vi "Get Sciscan Scope Image Equalization.vi"(0 "GFG Refnum":refnum<vi>, 5 "error in":errorcluster) -> (14 "GFG Refnum Out":refnum<vi>, 15 "Green Channel":cluster{dbl, dbl}(slide)={0.0, 7.070707070707071} caption="Green Channel Equalizer" scale=-32768.0..32767.0, 16 "Auto Adjust Green":bool, 17 "Red Channel":cluster{dbl, dbl}(slide)={0.0, 7.070707070707071} caption="Green Channel Equalizer" scale=-32768.0..32767.0, 18 "Auto Adjust Red":bool, 19 "error out":errorcluster)   [LabVIEW 2012, in "Sciscan Scope Daemon.lvlib"]
uses:
  Sciscan Scope Daemon.lvlib
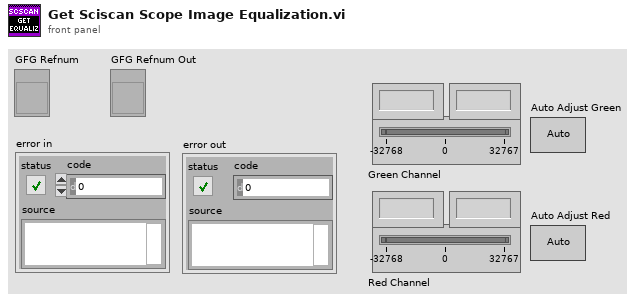
[diagram p1: front panel]
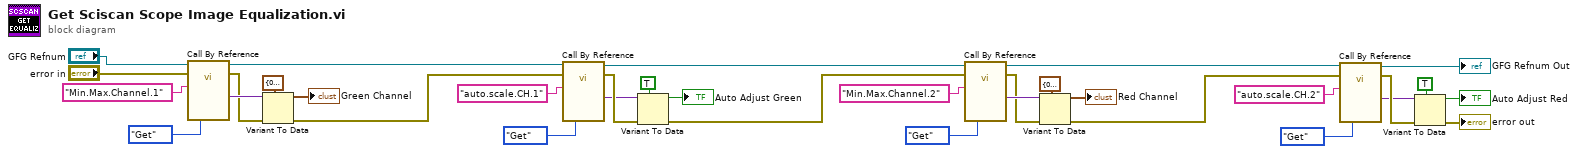
[diagram p0: block diagram]
diagram:
  n1 = call-by-ref "?"(reference="GFG Refnum", error in="error in", "Variable Name in"="Min.Max.Channel.1", "Action"=enum16{"Init", "Set", "Get"}."Get") -> (reference out=w26:refnum<vi>, error out=w27:errorcluster, "Variant Out"=w29:variant)  [unwired: 11 in, 6 out]
  n2 = Variant To Data(error in=w27, type=cluster{dbl, dbl} {0.0, 0.0} ("Green Channel"), Variant=w29) -> (data=→"Green Channel":cluster{dbl, dbl}, error out=w25:errorcluster)
  n3 = call-by-ref "?"(reference=w26, error in=w25, "Variable Name in"="auto.scale.CH.1", "Action"=enum16{"Init", "Set", "Get"}."Get") -> (reference out=w5:refnum<vi>, error out=w33:errorcluster, "Variant Out"=w32:variant)  [unwired: 11 in, 6 out]
  n4 = Variant To Data(error in=w33, type=TRUE, Variant=w32) -> (data=→"Auto Adjust Green":bool, error out=w4:errorcluster)
  n5 = call-by-ref "?"(reference=w5, error in=w4, "Variable Name in"="Min.Max.Channel.2", "Action"=enum16{"Init", "Set", "Get"}."Get") -> (reference out=w11:refnum<vi>, error out=w12:errorcluster, "Variant Out"=w14:variant)  [unwired: 11 in, 6 out]
  n6 = Variant To Data(error in=w12, type=cluster{dbl, dbl} {0.0, 0.0} ("Green Channel"), Variant=w14) -> (data=→"Red Channel":cluster{dbl, dbl}, error out=w10:errorcluster)
  n7 = call-by-ref "?"(reference=w11, error in=w10, "Variable Name in"="auto.scale.CH.2", "Action"=enum16{"Init", "Set", "Get"}."Get") -> (reference out=→"GFG Refnum Out":refnum<vi>, error out=w18:errorcluster, "Variant Out"=w17:variant)  [unwired: 11 in, 6 out]
  n8 = Variant To Data(error in=w18, type=TRUE, Variant=w17) -> (data=→"Auto Adjust Red":bool, error out=→"error out":errorcluster)
